vi "Write_RFID.vi"(8 "error in (no error)":errorcluster) -> (0 "error out":errorcluster)   [LabVIEW 2020]
uses:
  Sub VIs/MS SQL/MS_Global.vi
  <vilib>/ethernetip/ethernetip.llb/EthernetIP Tag Write BOOL.vi
  <vilib>/addons/database/_DB Variant To Data/Database Variant To Data.xnode
  <vilib>/addons/database/NI_Database_API.lvlib
  <vilib>/ethernetip/ethernetip.lvlib
panel:
  out "RFID@OP10":string
  in  "Write":bool
  in  "Refresh":bool
  in  "Pokayoke RFID":u16(ring) items=["PKYK00001C13", "PKYK00002C13", "PKYK00003C13", "PKYK00004C13", "PKYK00005C13", "PKYK00006C13", "PKYK00007C13", "PKYK00008C13"]
  # "PKYK RFID Generator"
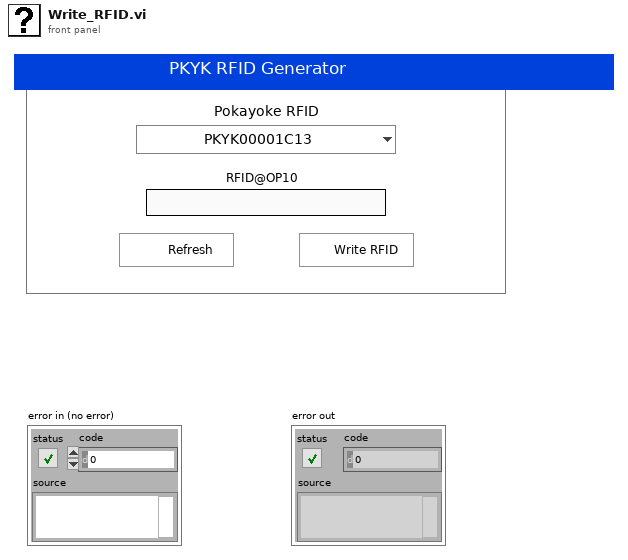
[diagram p1: front panel]
types:
  T1 = cluster{"Calibration":bool, "Settings":bool, "Script":bool, "Desktop Report":bool, "Help":bool}
  T2 = typedef "TD SQL.ctl" = cluster{"MS SQL Connection":T3, "UDL File":path, "Time":string, "DCODE":string, "WIP+1":i64, "MC No?":i32, "POKAYOKE?":bool, "Expected Result":string, "Result [Status]":string, "Clock":dbl, "RFID":string, "WIP Queue":refnum<queue>, "TS Parameter":T4, "Data_Queue":refnum<queue>[], "RFID Serial No.":string}
  T3 = typedef "NI_Database_API.lvlib/Conn ObjectReference.ctl" = refnum<k1>
  T4 = typedef "TS_Parameter.ctl" = cluster{"ProfitCenterCode":string, "LineCode":string, "WorkOrderNumber":string, "Model":string, "Model_with_Prefix":string, "VendorCode":string, "SetParameterDateCode":string, "PokaYoke":i32, "Target":i32, "Live_DateCode":string, "CustomerPartNumber":string, "Hand":string, "sBarcode":bool, "FCA":i32, "Ent_Stamp":timestamp, "STS_CD":dbl}
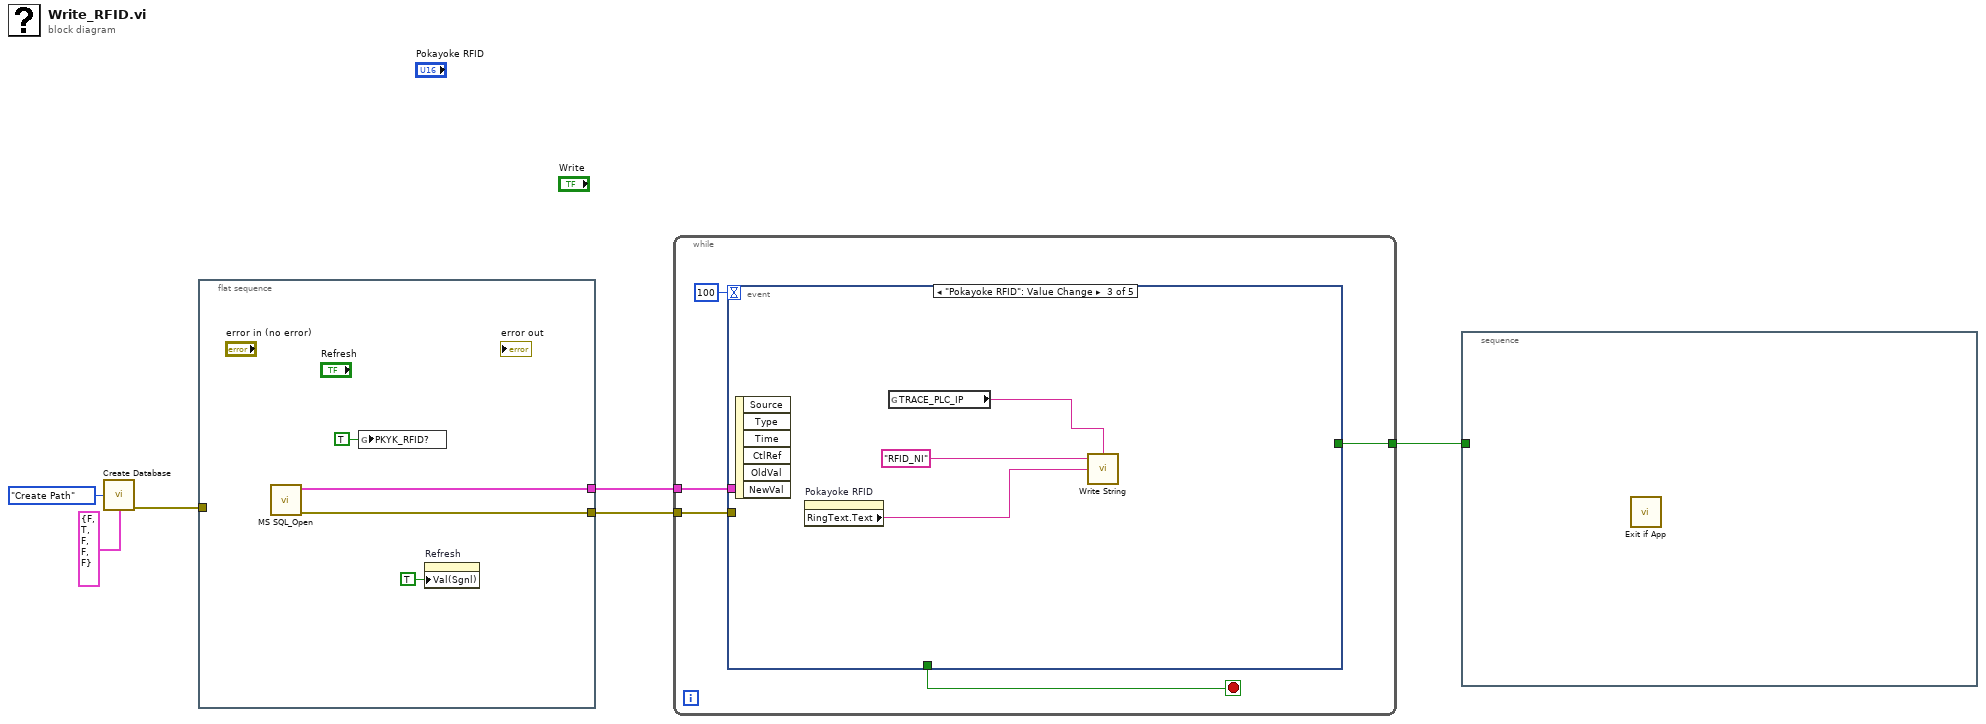
[diagram p0: block diagram]
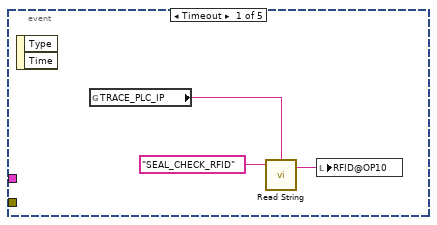
[diagram p2: hidden frame]
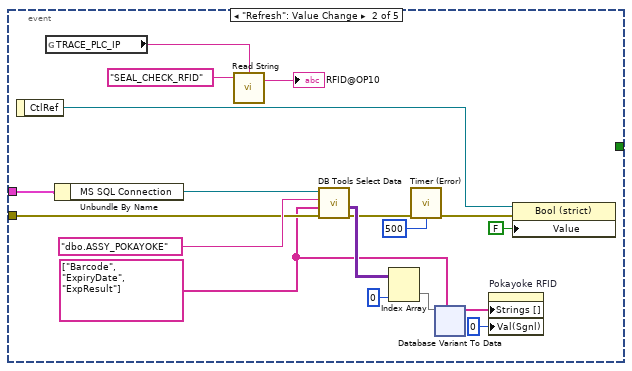
[diagram p3: hidden frame]
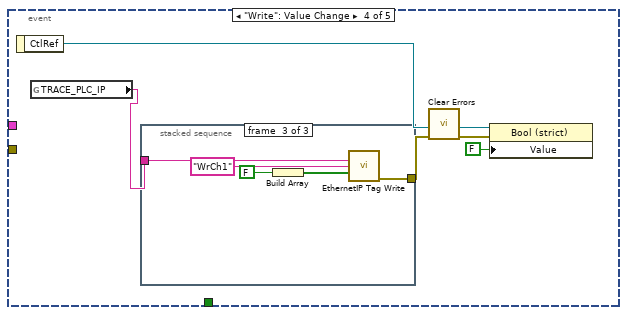
[diagram p4: hidden frame]
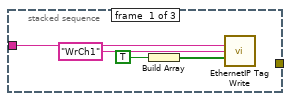
[diagram p5: hidden frame]
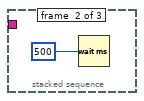
[diagram p6: hidden frame]
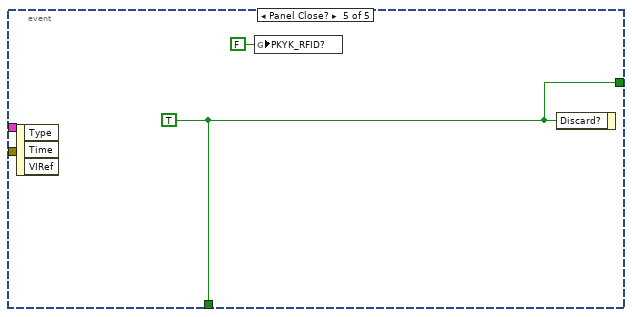
[diagram p7: hidden frame]
diagram:
  n1 = call <userlib>:"Create Database.vi"("Get/Create"=enum16{"Get Path", "Create Path"}."Create Path", "Create Folder"=T1 {"Calibration"=FALSE, "Settings"=TRUE, "Script"=FALSE, "Desktop Report"=FALSE, "Help"=FALSE}) -> ("error out"=w2:errorcluster)  [unwired: 12 in, 1 out]
  n2 = flat-sequence {
    tunnel: [w10] -> w6
    tunnel: [w9] -> w5
    tunnel: w2 -> [_]
    frame #0 {
      n3 = call "MS SQL_Open.vi"() -> ("error out"=w9:errorcluster, "Ref Out"=w10:T2)  [unwired: 9 in, 1 out]
      n4 = global write "MS_Global.vi" "PKYK_RFID?"(TRUE ("PKYK_RFID?")) -> ()
      n5 = property on="Refresh" class="Bool (strict)"("Val(Sgnl)"=TRUE ("Value (Signaling)")) -> ()  [unwired: 2 in, 2 out]
    }
  }
  n6 = while {
    tunnel: w6 -> [w14]
    tunnel: w5 -> [w13]
    tunnel: [w11] -> w4
    stop <- w15 stop-if-true
    n7 = event shown="[2] \"Pokayoke RFID\": Value Change" {
      selector: _ -> [_ _ _ _ _]
      dyn-events: _ -> [_ _ _ _ _]
      timeout: 100 -> [_ _ _ _ _]
      tunnel: [_ _ _ _ w93] -> w15
      tunnel: w14 -> [_ w34 _ _ _]
      tunnel: w13 -> [_ w33 _ _ _]
      tunnel: [_ _ _ _ w93] -> w11
      event Timeout {
        n8 = event-data() -> ()  [unwired: 1 in, 2 out]
        n9 = global read "MS_Global.vi" "TRACE_PLC_IP"() -> (w16:string)
        n10 = call "Read String.vi"("Network Path"=w16, "Tag Name"="SEAL_CHECK_RFID") -> ("String"=w18:string)  [unwired: 3 in]
        n11 = local write "RFID@OP10"(w18) -> ()
      }
      event "Refresh": Value Change {
        w30 = string[] ["Barcode", "ExpiryDate", "ExpResult"] ("columns")
        n12 = event-data() -> ("CtlRef"=w27:refnum<vi>)  [unwired: 1 in]
        n13 = global read "MS_Global.vi" "TRACE_PLC_IP"() -> (w19:string)
        n14 = Unbundle By Name(w34) -> ("MS SQL Connection"=w35:T3)
        n15 = call "Read String.vi"("Network Path"=w19, "Tag Name"="SEAL_CHECK_RFID") -> ("String"=→"RFID@OP10":string)  [unwired: 3 in]
        n16 = call <vilib>:"DB Tools Select Data.vi"("error in (no error)"=w33, "columns"=w30, "table"="dbo.ASSY_POKAYOKE", "connection reference"=w35) -> ("error out"=w26:errorcluster, "data"=w32:variant[][])  [unwired: 2 in, 1 out]
        n17 = Index Array(array=w32, index (col)=0 ("index (row)")) -> (element=w31:variant[])  [unwired: 1 in]
        n18 = call <userlib>:"Timer (Error).vi"("error in (no error)"=w26, "milliseconds to wait"=u32 500) -> ("error out"=w24:errorcluster)  [unwired: 13 in]
        n19 = xnode "Database Variant To Data"("database variant"=w31, "type"=w30) -> ("data"=w29:string[])  [unwired: 1 in, 1 out]
        n20 = property on="Pokayoke RFID" class="Ring (strict)"("Strings []"=w29, "Val(Sgnl)"=u16 0 ("Value (Signaling)")) -> ()  [unwired: 2 in, 2 out]
        n21 = property class="Bool (strict)"(reference=w27, error in=w24, "Value"=FALSE) -> ()  [unwired: 2 out]
      }
      event "Pokayoke RFID": Value Change {
        n22 = event-data() -> ()  [unwired: 1 in, 6 out]
        n23 = property on="Pokayoke RFID" class="Ring (strict)"() -> ("RingText.Text"=w76:string)  [unwired: 2 in, 2 out]
        n24 = global read "MS_Global.vi" "TRACE_PLC_IP"() -> (w75:string)
        n25 = call "Write String.vi"("Network Path"=w75, "String"=w76, "Tag Name"="RFID_NI" ("Data")) -> ()  [unwired: 2 in]
      }
      event "Write": Value Change {
        n26 = event-data() -> ("CtlRef"=w82:refnum<vi>)  [unwired: 1 in]
        n27 = global read "MS_Global.vi" "TRACE_PLC_IP"() -> (w78:string)
        n28 = stacked-sequence {
          tunnel: w78 -> [w86 _ w92]
          tunnel: [_ _ w88] -> w81
          frame #0 {
            n29 = Build Array(TRUE) -> (w84:bool[])
            n30 = call-poly <vilib>:"EthernetIP Tag Write.vi"("Network Path"=w86, "Tag Name"="WrCh1", "Data"=w84) -> ()  [unwired: 11 in, 2 out]
          }
          frame #1 {
            n31 = Wait (ms)(milliseconds to wait=u32 500) -> ()  [unwired: 1 out]
          }
          frame #2 {
            n32 = Build Array(FALSE) -> (w90:bool[])
            n33 = call-poly <vilib>:"EthernetIP Tag Write.vi"("Network Path"=w92, "Tag Name"="WrCh1", "Data"=w90) -> ("error out"=w88:errorcluster)  [unwired: 11 in, 1 out]
          }
        }
        n34 = call <vilib>:"Clear Errors.vi"("error in (no error)"=w81) -> ("error out"=w80:errorcluster)  [unwired: 5 in, 1 out]
        n35 = property class="Bool (strict)"(reference=w82, error in=w80, "Value"=FALSE) -> ()  [unwired: 2 out]
      }
      event Panel Close? {
        w93 = TRUE ("Discard?")
        n36 = event-data() -> ()  [unwired: 1 in, 3 out]
        n37 = global write "MS_Global.vi" "PKYK_RFID?"(FALSE ("PKYK_RFID?")) -> ()
        n38 = event-data("Discard?"=w93) -> ()  [unwired: 1 in, 1 out]
      }
    }
  }
  n39 = stacked-sequence {
    tunnel: w4 -> [_]
    frame #0 {
      n40 = call <userlib>:"Exit if App.vi"() -> ()  [unwired: 11 in, 1 out]
    }
  }
